vi "read_attributes.vi"(8 "error in (no error)":errorcluster, 11 "GradientBoostingRegressor in":refnum<class "GradientBoostingRegressor.lvclass">) -> (0 "error out":errorcluster, 2 "attributes":T1, 3 "GradientBoostingRegressor out":refnum<class "GradientBoostingRegressor.lvclass">)   [LabVIEW 2020, in "GradientBoostingRegressor.lvclass"]
uses:
  GradientBoostingRegressor.lvclass
  Controls/gradient_boosting_regressor_attributes.ctl
  GradientBoostingRegressor.lvclass/GradientBoostingRegressor.ctl
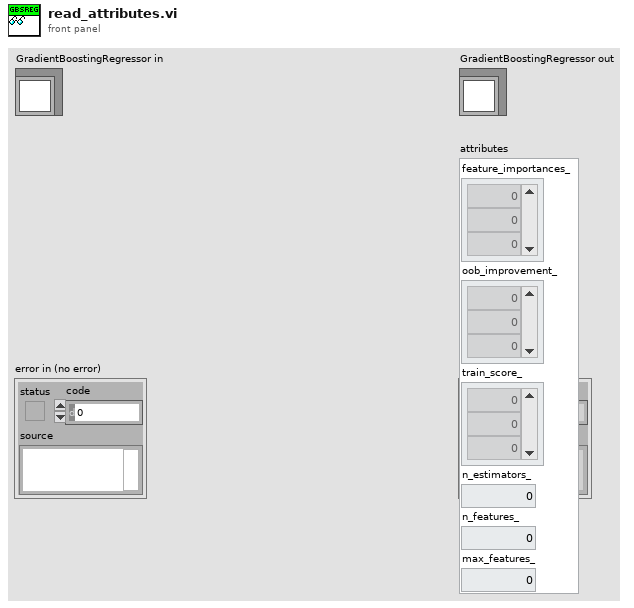
[diagram p1: front panel]
types:
  T1 = typedef "gradient_boosting_regressor_attributes.ctl" = cluster{"feature_importances_":dbl[], "oob_improvement_":dbl[], "train_score_":dbl[], "n_estimators_":dbl, "n_features_":dbl, "max_features_":dbl}
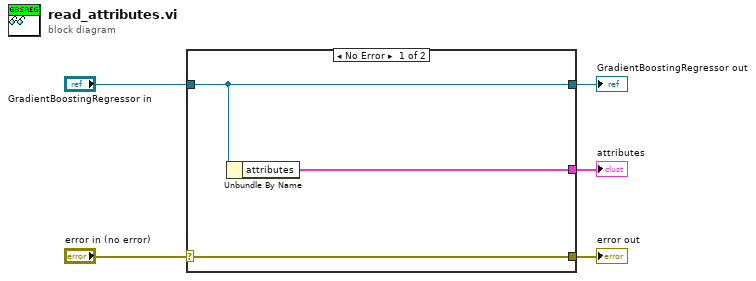
[diagram p0: block diagram]
diagram:
  n1 = case shown="No Error" "error in (no error)" {
    selector: "error in (no error)" -> [w8 w9]
    tunnel: [w8 w9] -> w4
    tunnel: [w7 w10] -> w2
    tunnel: "GradientBoostingRegressor in" -> [w7 w10]
    tunnel: [w6 _] -> w1
    frame No Error {
      n2 = Unbundle By Name(w7) -> ("attributes"=w6:T1)
    }
    frame Error {
    }
  }
  "error out" <- w4
  "GradientBoostingRegressor out" <- w2
  "attributes" <- w1
